vi "CleanUp.vi"(8 "error in (no error)":errorcluster, 11 "Prueba08 in":refnum<class "Prueba08.lvclass">) -> (0 "error out":errorcluster, 3 "Prueba08 out":refnum<class "Prueba08.lvclass">)   [LabVIEW 2019, in "Prueba08.lvclass"]
uses:
  Prueba08.lvclass
  C:/Users/ivan_/Documents/procal/Pruebas/Prueba/Prueba.lvclass
  Prueba/Prueba.lvclass/Prueba.ctl
  Prueba08.lvclass/Prueba08.ctl
  Base de Datos/SQLiteConnector/SQLiteConnection.lvclass
  Base de Datos/Base de Datos.lvclass
  Prueba/Prueba.lvclass
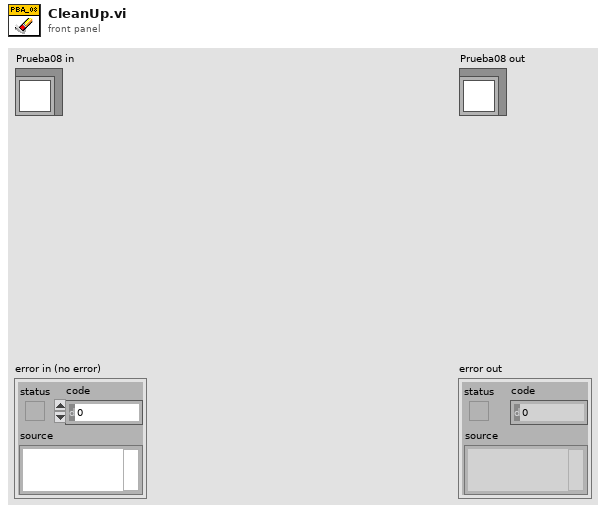
[diagram p1: front panel]
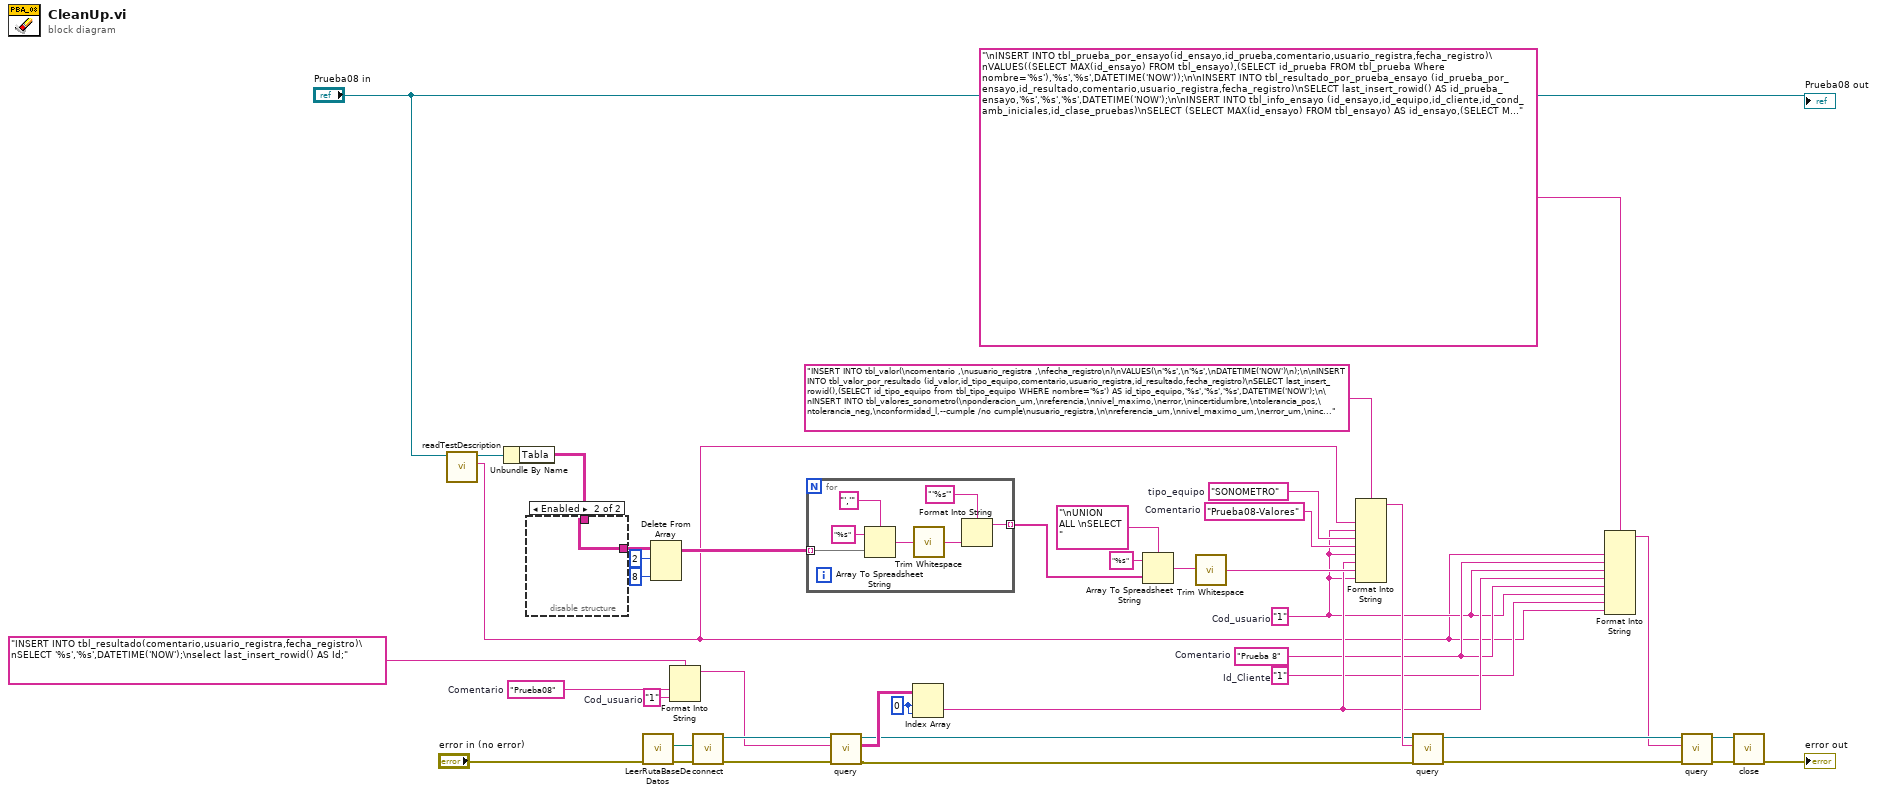
[diagram p0: block diagram]
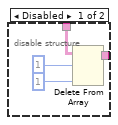
[diagram p2: hidden frame]
diagram:
  w13 = "1"  # Id_Cliente
  w14 = "Prueba 8"  # Comentario
  w23 = "SONOMETRO"  # tipo_equipo
  w22 = "Prueba08-Valores"  # Comentario
  w28 = 0 ("index (row)")
  w30 = "1"  # Cod_usuario
  w31 = "Prueba08"  # Comentario
  w12 = "1"  # Cod_usuario
  n1 = call "readTestDescription.vi"("Prueba in"="Prueba08 in") -> ("Test Description"=w4:string, "Prueba out"=w5:refnum<class "Prueba08.lvclass">)  [unwired: 8 in, 1 out]
  n2 = Unbundle By Name(w5) -> ("Tabla"=w7:string[][])
  n3 = disable-structure shown="Enabled" {
    disable-tunnel: [w44 w46] -> w9
    disable-tunnel: w7 -> [w43 w46]
    frame Disabled {
      n4 = Delete From Array(array=w43, length=1, index (col)=1 ("disabled index (col)")) -> (array with subset deleted=w44:string[][])  [unwired: 1 in, 1 out]
    }
    frame Enabled {
    }
  }
  n5 = call "LeerRutaBaseDeDatos.vi"("error in (no error)"="error in (no error)") -> ("error out"=w36:errorcluster, "Database Path"=w35:path)  [unwired: 9 in]
  n6 = Delete From Array(array=w9, length=2, index (col)=8 ("disabled index (col)")) -> (array with subset deleted=w10:string[][])  [unwired: 1 in, 1 out]
  n7 = Format Into String(format string="INSERT INTO tbl_resultado(comentario,usuario_registra,fecha_registro)\nSELECT '%s','%s',DATETIME('NOW');\nselect last_insert_rowid() AS Id;" ("SQL Statement"), w31, w30) -> (resulting string=w29:string)  [unwired: 2 in, 1 out]
  n8 = call "connect.vi"("error in (no error)"=w36, "Database Path"=w35) -> ("error out"=w27:errorcluster, "object out"=w33:refnum<class "SQLiteConnection.lvclass">)  [unwired: 8 in]
  n9 = for {
    tunnel: w10 -> [w47] mode=indexing
    tunnel: [w50] -> w39 mode=indexing
    n10 = Array To Spreadsheet String(delimiter (Tab)="','", array=w47, 3:"%s" ("format string")) -> (spreadsheet string=w49:string)
    n11 = call <vilib>:"Trim Whitespace.vi"("string"=w49) -> ("trimmed string"=w48:string)  [unwired: 1 in]
    n12 = Format Into String(format string="'%s'", w48) -> (resulting string=w50:string)  [unwired: 2 in, 1 out]
  }
  n13 = call "query.vi"("error in (no error)"=w27, "SQL Statement"=w29, "object in"=w33) -> ("error out"=w8:errorcluster, "result"=w26:string[][], "object out"=w25:refnum<class "SQLiteConnection.lvclass">)  [unwired: 5 in, 1 out]
  n14 = Index Array(array=w26, index (row)=w28, index (col)=w28) -> (element=w15:string)
  n15 = Array To Spreadsheet String(delimiter (Tab)="\nUNION ALL \nSELECT ", array=w39, 3:"%s" ("format string")) -> (spreadsheet string=w38:string)
  n16 = call <vilib>:"Trim Whitespace.vi"("string"=w38) -> ("trimmed string"=w24:string)  [unwired: 1 in]
  n17 = Format Into String(format string="INSERT INTO tbl_valor(\ncomentario ,\nusuario_registra ,\nfecha_registro\n)\nVALUES(\n'%s',\n'%s',\nDATETIME('NOW')\n);\n\nINSERT INTO tbl_valor_por_resultado (id_valor,id_tipo_equipo,comentario,usuario_registra,id_resultado,fecha_registro)\nSELECT last_insert_rowid(),(SELECT id_tipo_equipo from tbl_tipo_equipo WHERE nombre='%s') AS id_tipo_equipo,'%s','%s','%s',DATETIME('NOW');\n\nINSERT INTO tbl_valores_sonometro(\nponderacion_um,\nreferencia,\nnivel_maximo,\nerror,\nincertidumbre,\ntolerancia_pos,\ntolerancia_neg,\nconformidad_l,--cumple /no cumple\nusuario_registra,\n\nreferencia_um,\nnivel_maximo_um,\nerror_um,\nincertidumbre_um,\ntolerancia_pos_um,\ntolerancia_neg_um,\n\nid_valor,\nfecha_registro\n)\nSELECT * FROM(\nSELECT %s\n) AS T\nINNER JOIN\n(SELECT %s AS usuario,'dB','dB','dB','dB','dB','dB',(SELECT MAX(id_valor) FROM tbl_valor) AS id_valor,DATETIME('NOW') fecha ) AS F;\n", w4, w12, w23, w22, w12, w15, w24, w12) -> (resulting string=w34:string)  [unwired: 2 in, 1 out]
  n18 = call "query.vi"("error in (no error)"=w8, "SQL Statement"=w34, "object in"=w25) -> ("error out"=w19:errorcluster, "object out"=w21:refnum<class "SQLiteConnection.lvclass">)  [unwired: 5 in, 2 out]
  n19 = Format Into String(format string="\nINSERT INTO tbl_prueba_por_ensayo(id_ensayo,id_prueba,comentario,usuario_registra,fecha_registro)\nVALUES((SELECT MAX(id_ensayo) FROM tbl_ensayo),(SELECT id_prueba FROM tbl_prueba Where nombre='%s'),'%s','%s',DATETIME('NOW'));\n\nINSERT INTO tbl_resultado_por_prueba_ensayo (id_prueba_por_ensayo,id_resultado,comentario,usuario_registra,fecha_registro)\nSELECT last_insert_rowid() AS id_prueba_ensayo,'%s','%s','%s',DATETIME('NOW');\n\nINSERT INTO tbl_info_ensayo (id_ensayo,id_equipo,id_cliente,id_cond_amb_iniciales,id_clase_pruebas)\nSELECT (SELECT MAX(id_ensayo) FROM tbl_ensayo) AS id_ensayo,(SELECT MAX(id_equipo) FROM tbl_equipo) AS id_equipo,'%s' AS id_cliente,(SELECT MAX(id_cond_amb_iniciales) FROM tbl_cond_amb_iniciales) AS id_cond_amb_iniciales,\n(SELECT id_clase_prueba FROM tbl_clase_prueba WHERE id_clase=(SELECT id_clase FROM tbl_equipo ORDER BY id_equipo DESC LIMIT 1)  AND id_prueba=(SELECT id_prueba FROM tbl_prueba Where nombre='%s')) AS id_clase_pruebas;\n", w4, w14, w12, w15, w14, w12, w13, w4) -> (resulting string=w16:string)  [unwired: 2 in, 1 out]
  n20 = call "query.vi"("error in (no error)"=w19, "SQL Statement"=w16, "object in"=w21) -> ("error out"=w18:errorcluster, "object out"=w20:refnum<class "SQLiteConnection.lvclass">)  [unwired: 5 in, 2 out]
  n21 = call-dynamic "close.vi"("error in (no error)"=w18, "object in"=w20) -> ("error out"=→"error out":errorcluster)  [unwired: 8 in, 1 out]
  "Prueba08 out" <- "Prueba08 in"
